vi "Slice Engine.vi"(8 "error in (no error)":errorcluster, 10 "Slice thickness  (mm)":dbl=150.0, 11 "System Parameters":T1={"Vibratome"={"Z Bottom [mm]"=0.0, "Pre Cut Dwell [s]"=1.0, "Blade Frequency [RPM]"=3000, "Slice Speed [mm/s]"=0.1, "Post Cut Dwell [s]"=4.0, "Ramp Time [s]"=0.5, "Start X [mm]"=80.5, "Start Y [mm]"=72.0, "Slice Length [mm]"=15.0, "Slice Axis"=enum."X Axis", "Controller VISA Ref"="COM3"}, "Table Stages"={"X Stage"={"Position"=0.0, "Is.Enabled?"=FALSE, "Is.Connected?"=FALSE, "Device SN"="45876060", "AccelerationMaximum"=50.0, "VelocityMaximum"=50.0, "Acceleration"=20.0, "Velocity"=20.0, "waitTimeout (ms)"=1000000, "Model"=enum."Thorlabs LTS", "Is.Homed?"=FALSE}, "Y Stage"={"Position"=0.0, "Is.Enabled?"=FALSE, "Is.Connected?"=FALSE, "Device SN"="45875512", "AccelerationMaximum"=50.0, "VelocityMaximum"=50.0, "Acceleration"=20.0, "Velocity"=20.0, "waitTimeout (ms)"=1000000, "Model"=enum."Thorlabs LTS", "Is.Homed?"=FALSE}, "Z Stage"={"Position"=0.0, "Is.Enabled?"=FALSE, "Is.Connected?"=FALSE, "Device SN"="49872414", "AccelerationMaximum"=50.0, "VelocityMaximum"=50.0, "Acceleration"=20.0, "Velocity"=20.0, "waitTimeout (ms)"=100000, "Model"=enum."Thorlabs MLJ", "Is.Homed?"=FALSE}}}) -> (0 "error out":errorcluster)   [LabVIEW 2017]
uses:
  Controls/System Parameters.ctl
  Hardware/Table Stage/Controls/Translation Stage Cluster.ctl
  Controls/Translation Stage Types.ctl
  Controls/Queue Manager Actions.ctl
  Controls/QueueNames.ctl
  Hardware/Table Stage/Controls/Motion Translation Module Control.ctl
  Controls/Set Get Controls.ctl
panel:
  in  "Last Slice?":bool
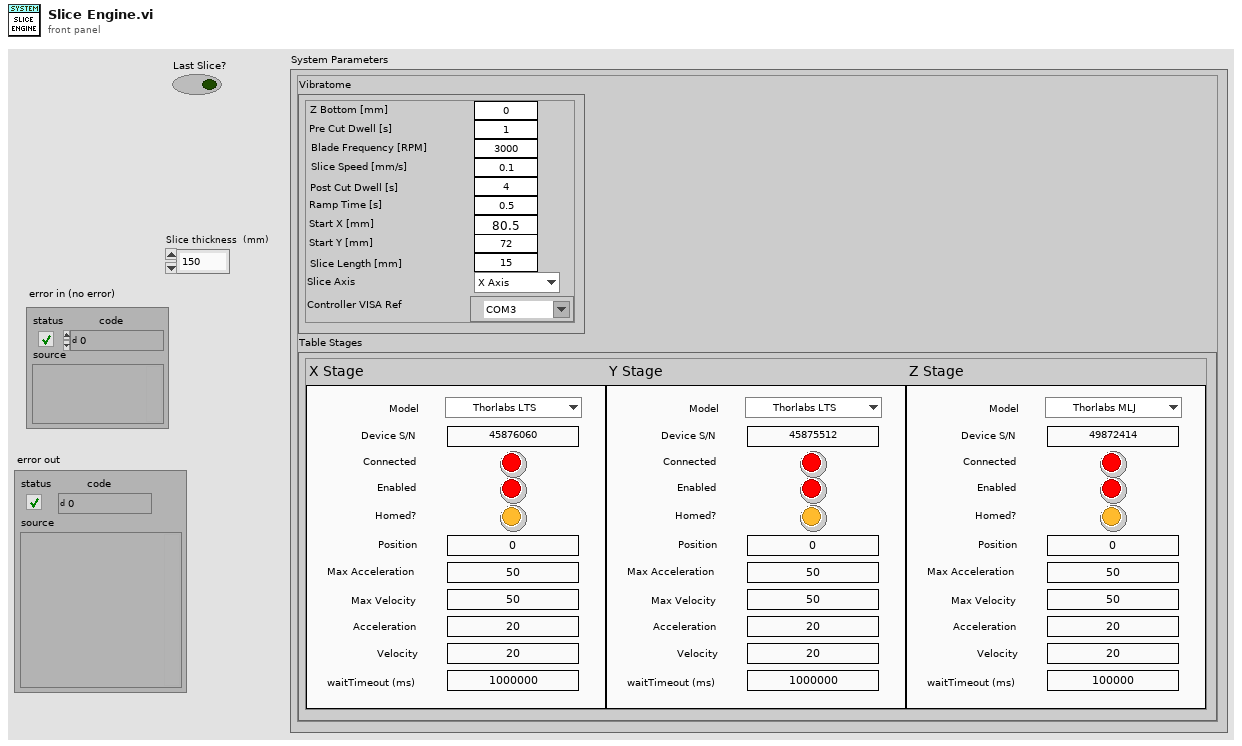
[diagram p1: front panel]
types:
  T1 = typedef "System Parameters.ctl" = cluster{"Vibratome":cluster{"Z Bottom [mm]":dbl, "Pre Cut Dwell [s]":dbl, "Blade Frequency [RPM]":u16, "Slice Speed [mm/s]":dbl, "Post Cut Dwell [s]":dbl, "Ramp Time [s]":dbl, "Start X [mm]":dbl, "Start Y [mm]":dbl, "Slice Length [mm]":dbl, "Slice Axis":enum16{"X Axis", "Y Axis", "Z Axis"}, "Controller VISA Ref":refnum<visa-resource-name>}, "Table Stages":cluster{"X Stage":T2, "Y Stage":T2, "Z Stage":T2}}
  T2 = typedef "Translation Stage Cluster.ctl" = cluster{"Position":dbl, "Is.Enabled?":bool, "Is.Connected?":bool, "Device SN":string, "AccelerationMaximum":dbl, "VelocityMaximum":dbl, "Acceleration":dbl, "Velocity":dbl, "waitTimeout (ms)":i32, "Model":T3, "Is.Homed?":bool}
  T3 = typedef "Translation Stage Types.ctl" = enum16{"None", "Thorlabs LTS", "Thorlabs MLJ"}
  T4 = typedef "QueueNames.ctl" = enum16{"Main GUI", "Main Scan Processor", "Main Display", "Main Table Stage GUI", "Main Table Stage Proc.", "Scan Engine", "Vibratome GUI", "Vibratome Processor", "Slice Engine"}
  T5 = typedef "Queue Manager Actions.ctl" = enum16{"Init", "Enqueue", "Enqueue All", "Preview Queue", "Dequeue", "Get Status", "Flush Queue", "Flush All Queues", "Release All Queues", "Release Queue", "Enqueue at Opposite End"}
  T6 = typedef "Set Get Controls.ctl" = enum16{"Set", "Get"}
  T7 = typedef "Motion Translation Module Control.ctl" = enum16{"Init", "Home", "Status", "Velocity/Accel", "Position", "Jog", "Stop", "Uninit", "Enable", "Disable"}
  T8 = enum16{"Set Configuration", "Get Configuration", "Enable Motor", "Disable Motor", "Get Status", "Open Session", "Close Session", "Set Limits", "Get Limits"}
  T9 = cluster{"Source for Velocity":enum16{"Interface", "Voltage (AI)", "PWM (AI)", "Current Target (AI)", "Current Target w/ Preset (AI)"}, "Mode":enum16{"Continuous", "Stepper Motor", "Analog Position Ctrl", "Encoder"}, "Target Velocity [RPM]":i16}
  T10 = typedef "MessagePacket.ctl" = cluster{"Message":string, "Parameter":variant}
  T11 = cluster{"X Stage":T2, "Y Stage":T2, "Z Stage":T2}
  T12 = enum16{"Left Button", "Center Button", "Right Button", "Window Close"}
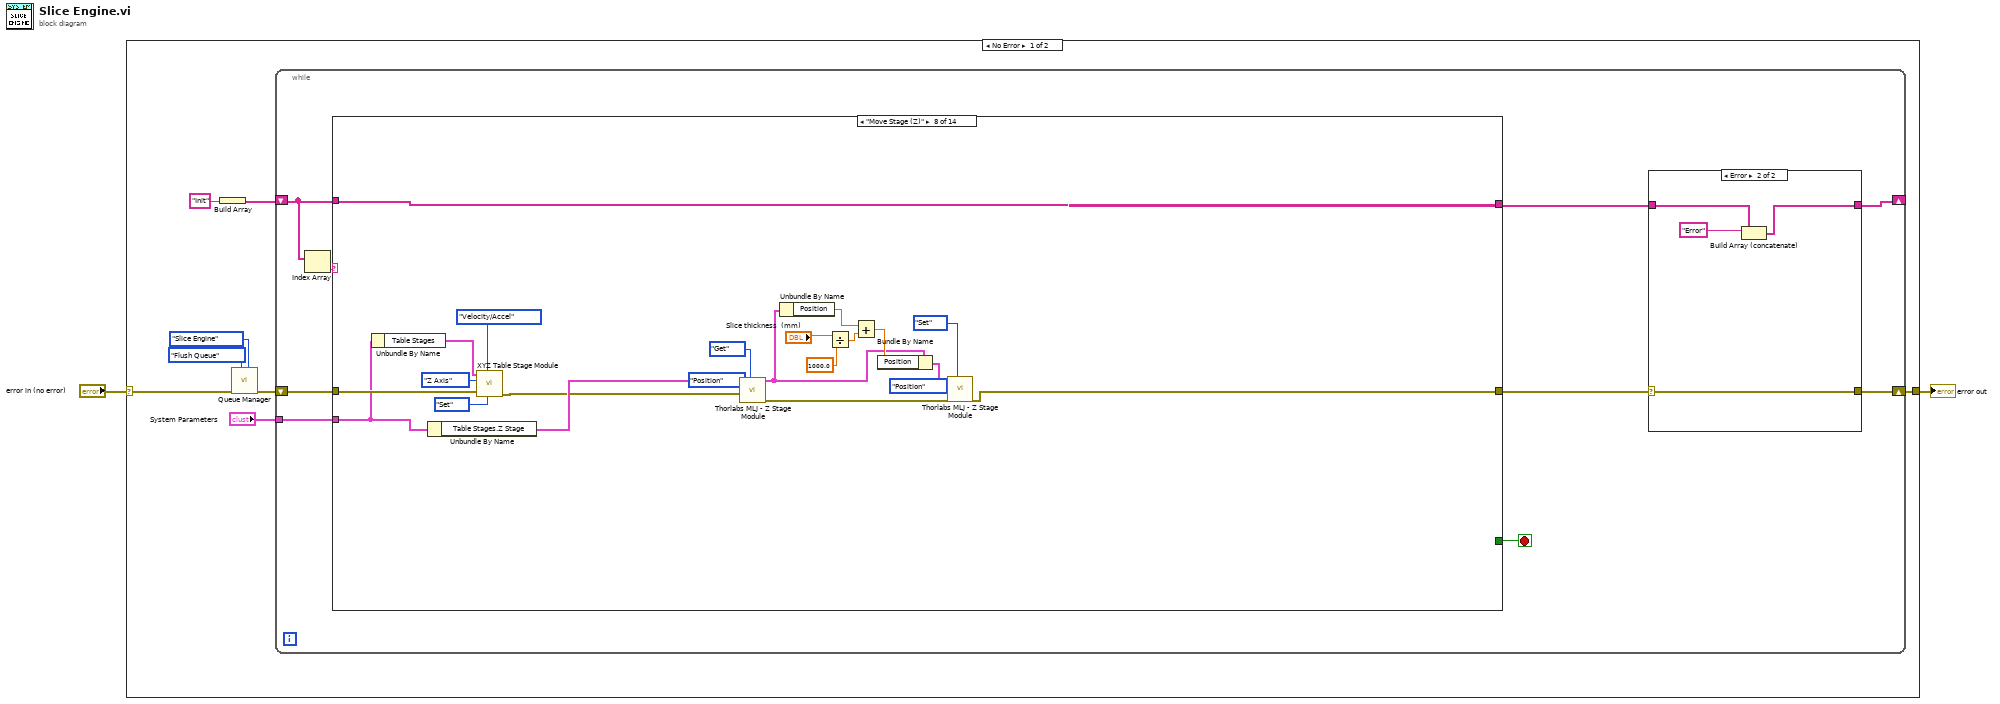
[diagram p0: block diagram]
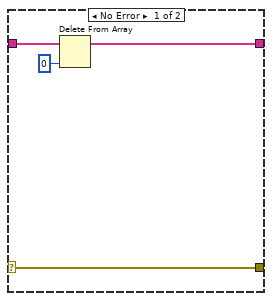
[diagram p2: hidden frame]
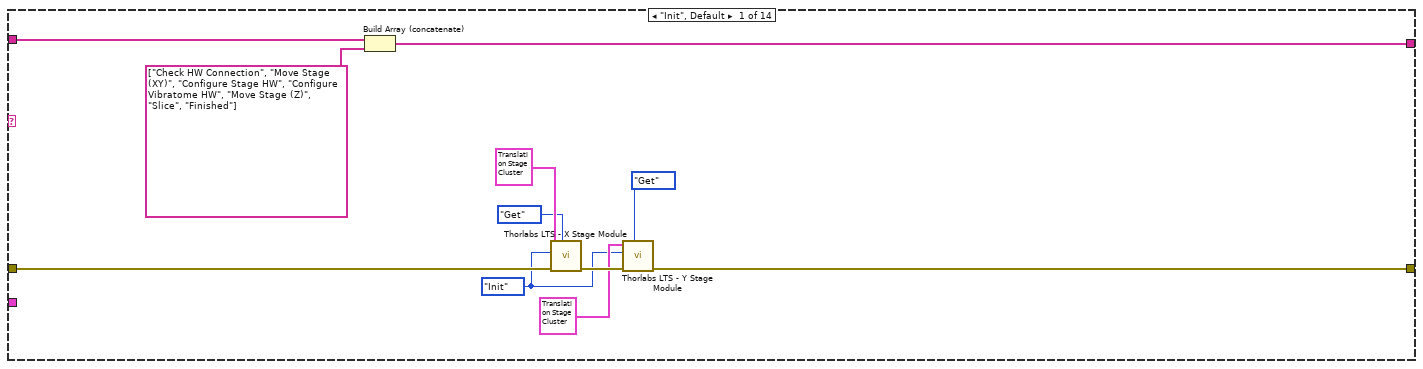
[diagram p3: hidden frame]
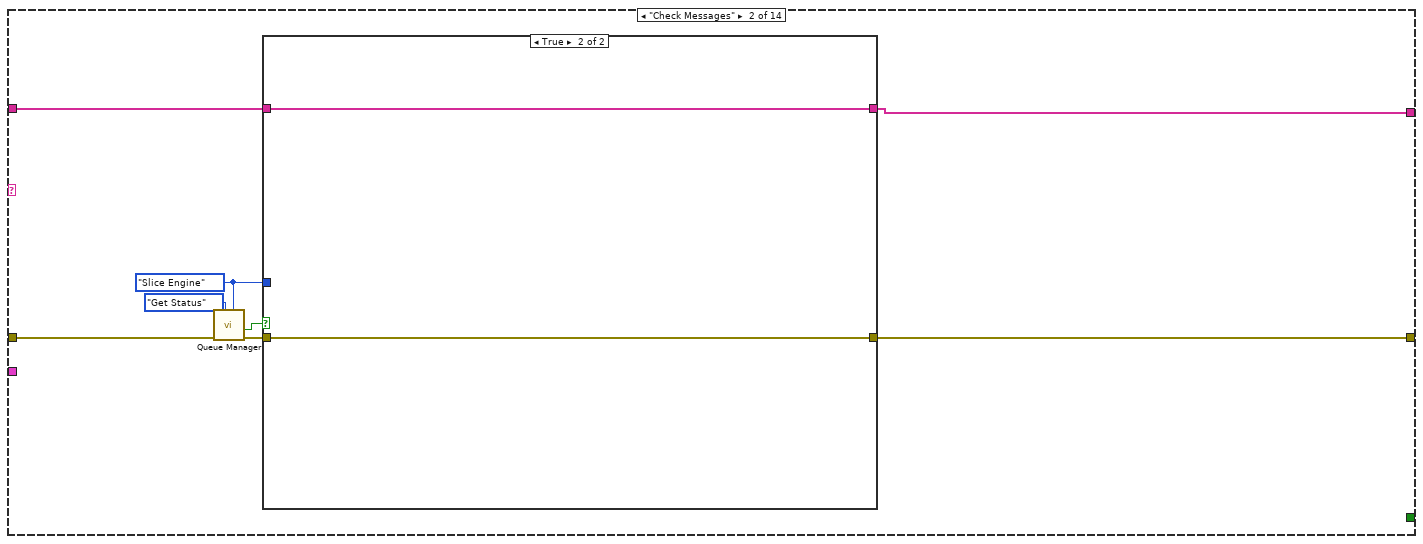
[diagram p4: hidden frame]
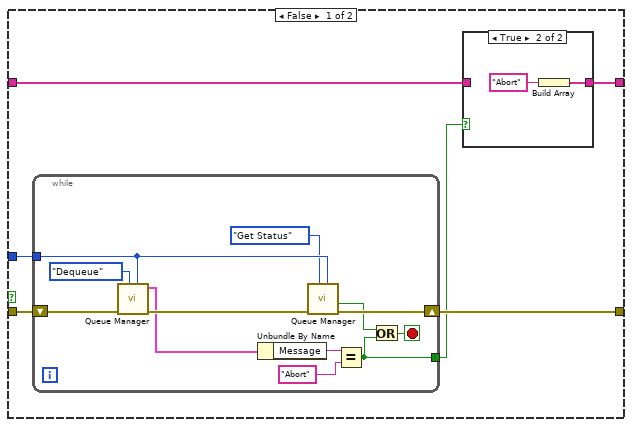
[diagram p5: hidden frame]
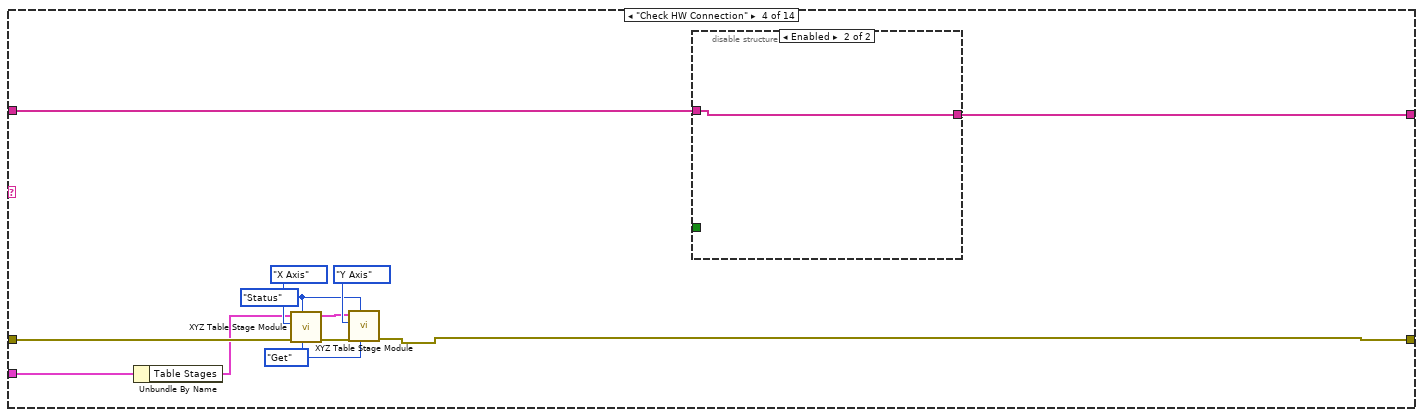
[diagram p8: hidden frame]
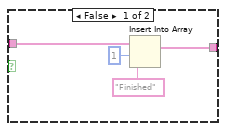
[diagram p10: hidden frame]
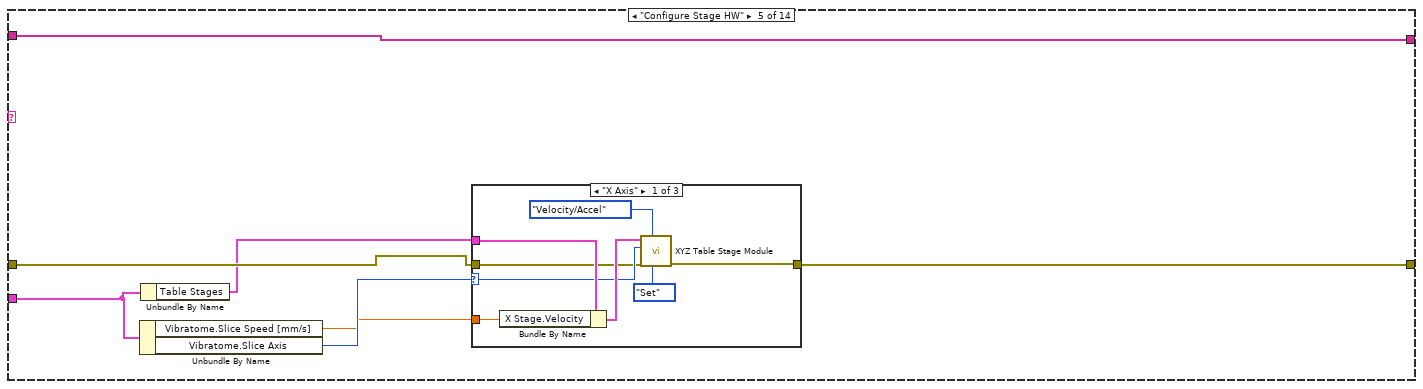
[diagram p11: hidden frame]
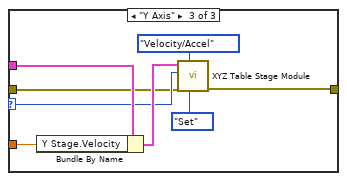
[diagram p13: hidden frame]
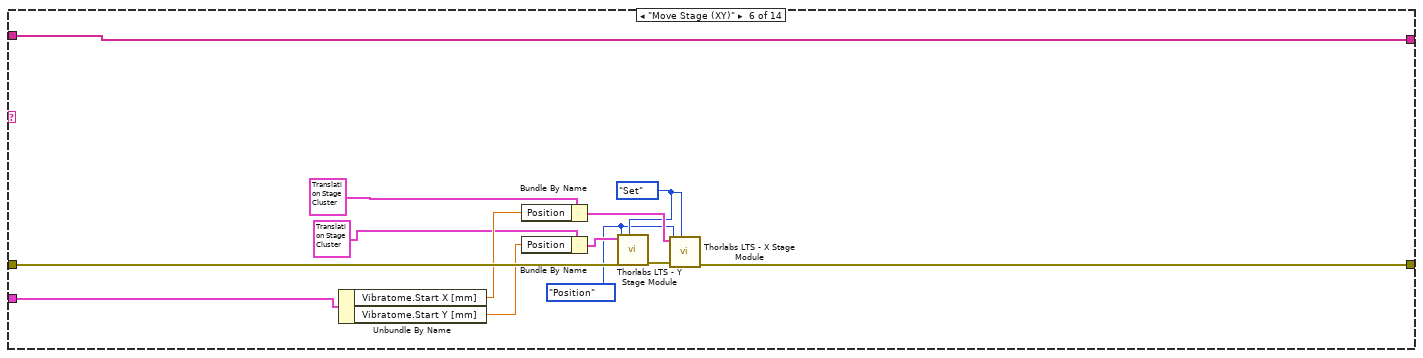
[diagram p14: hidden frame]
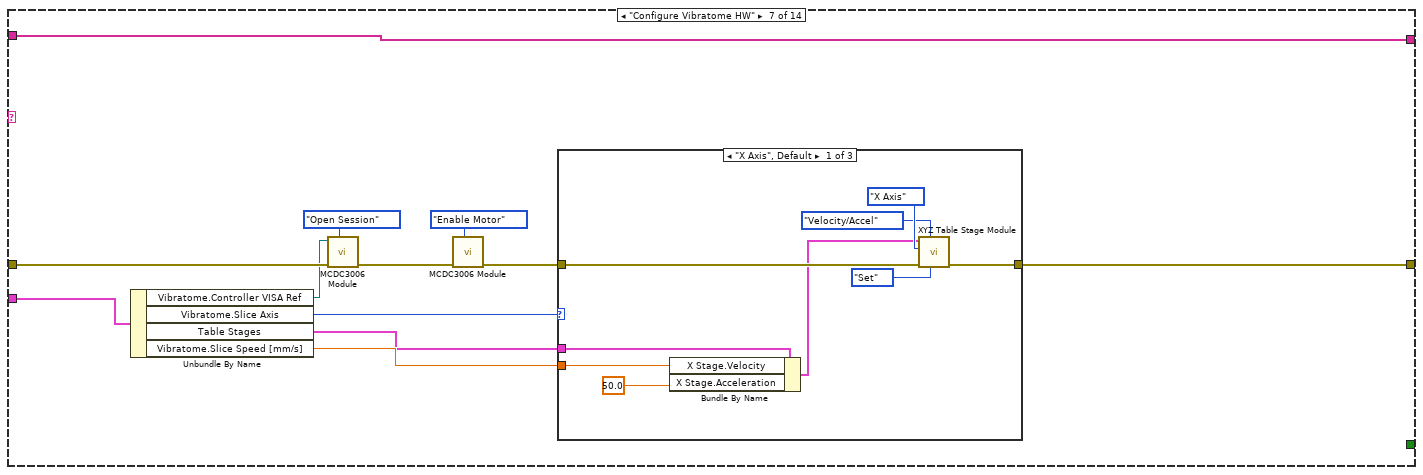
[diagram p15: hidden frame]
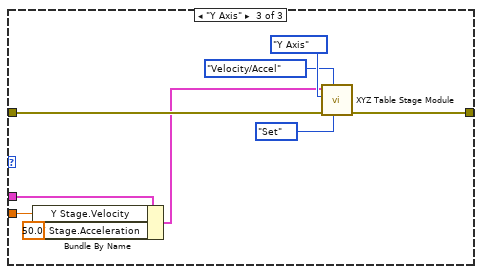
[diagram p17: hidden frame]
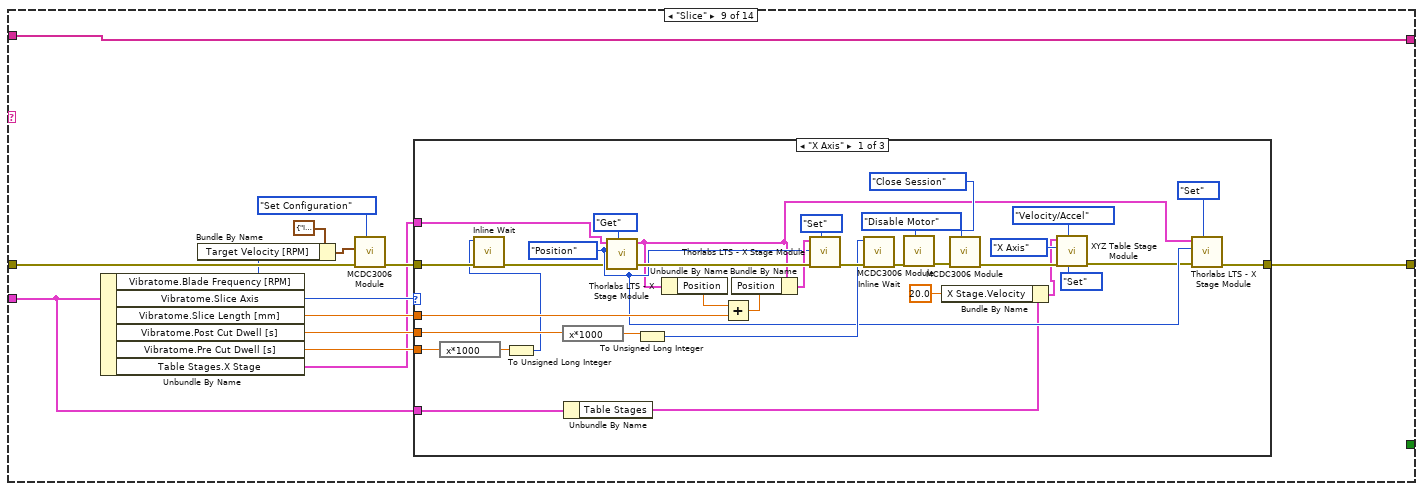
[diagram p18: hidden frame]
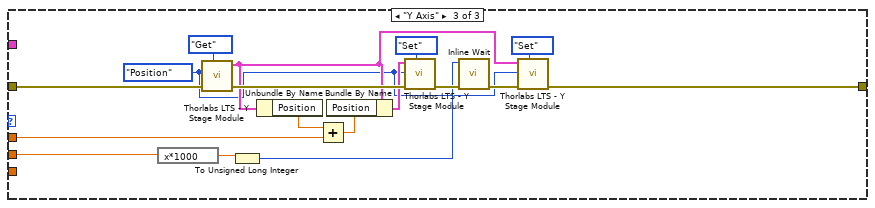
[diagram p20: hidden frame]
diagram:
  n1 = case shown="No Error" "error in (no error)" {
    selector: "error in (no error)" -> [w3 w392]
    tunnel: [w5 w392] -> w1
    frame No Error {
      n2 = Build Array("Init") -> (w6:string[])
      n3 = call "Queue Manager.vi"("Queue Name"=QueueNames."Slice Engine", "Action"=Queue_Manager_Actions."Flush Queue", "Error In"=w3) -> ("Error Out"=w9:errorcluster)  [unwired: 4 in, 4 out]
      n4 = while {
        shift-right: [w13] -> _
        shift-left: w6 -> [w12]
        shift-right: [w15] -> w5
        shift-left: w9 -> [w19]
        tunnel: "System Parameters" -> [w11]
        stop <- w17 stop-if-true
        n5 = Index Array(array=w12) -> (element=w18:string)  [unwired: 1 in]
        n6 = case shown="\"Move Stage (Z)\"" w18 {
          tunnel: w19 -> [w35 w46 w70 w83 w94 w129 w139 w167 w195 w249 w263 w267 w296 w365]
          tunnel: w12 -> [w38 w40 w71 w73 w99 w126 w141 w182 w194 w252 w260 w265 w297 w372]
          tunnel: [w37 w39 w71 w74 w99 w126 w141 w182 w194 w251 w261 w264 w297 w372] -> w14
          tunnel: [_ _ _ _ _ _ _ _ _ _ _ _ _ w371] -> w17
          tunnel: [w34 w41 w70 w72 w95 w128 w133 w176 w196 w249 w263 w268 w294 w363] -> w16
          tunnel: w11 -> [_ _ _ w82 w98 w127 w140 w163 w183 _ _ _ w295 w367]
          frame "Init", Default {
            w30 = Motion_Translation_Module_Control."Init" ("Action")
            n7 = Build Array (concatenate)(w38, string[] ["Check HW Connection", "Move Stage (XY)", "Configure Stage HW", "Configure Vibratome HW", "Move Stage (Z)", "Slice", "Finished"]) -> (w37:string[])
            n8 = call "Thorlabs LTS - X Stage Module.vi"("Set/Get"=Set_Get_Controls."Get", "Error In"=w35, "Action"=w30, "Cluster In"=T2 {"Position"=0.0, "Is.Enabled?"=TRUE, "Is.Connected?"=FALSE, "Device SN"="45876060", "AccelerationMaximum"=0.0, "VelocityMaximum"=0.0, "Acceleration"=0.0, "Velocity"=0.0, "waitTimeout (ms)"=10000, "Model"=enum."None", "Is.Homed?"=FALSE}) -> ("Error Out"=w33:errorcluster)  [unwired: 6 in, 1 out]
            n9 = call "Thorlabs LTS - Y Stage Module.vi"("Set/Get"=Set_Get_Controls."Get", "Error In"=w33, "Action"=w30, "Cluster In"=T2 {"Position"=0.0, "Is.Enabled?"=TRUE, "Is.Connected?"=FALSE, "Device SN"="45875512", "AccelerationMaximum"=0.0, "VelocityMaximum"=0.0, "Acceleration"=0.0, "Velocity"=0.0, "waitTimeout (ms)"=10000, "Model"=enum."None", "Is.Homed?"=FALSE}) -> ("Error Out"=w34:errorcluster)  [unwired: 6 in, 1 out]
          }
          frame "Check Messages" {
            w42 = QueueNames."Slice Engine" ("Queue Name")
            n10 = call "Queue Manager.vi"("Queue Name"=w42, "Action"=Queue_Manager_Actions."Get Status", "Error In"=w46) -> ("Error Out"=w43:errorcluster, "Empty?"=w44:bool)  [unwired: 4 in, 3 out]
            n11 = case shown="True" w44 {
              tunnel: w43 -> [w52 w68]
              tunnel: w42 -> [w51 _]
              tunnel: [w50 w68] -> w41
              tunnel: w40 -> [w48 w69]
              tunnel: [w47 w69] -> w39
              frame False {
                n12 = while {
                  tunnel: w51 -> [w63]
                  shift-right: [w64] -> w50
                  shift-left: w52 -> [w67]
                  tunnel: [w56] -> w49
                  stop <- w57 stop-if-true
                  n13 = call "Queue Manager.vi"("Queue Name"=w63, "Action"=Queue_Manager_Actions."Dequeue", "Error In"=w67) -> ("Error Out"=w65:errorcluster, "Message Packet [Out]"=w61:T10)  [unwired: 4 in, 3 out]
                  n14 = Unbundle By Name(w61) -> ("Message"=w60:string)
                  n15 = call "Queue Manager.vi"("Queue Name"=w63, "Action"=Queue_Manager_Actions."Get Status", "Error In"=w65) -> ("Error Out"=w64:errorcluster, "Empty?"=w58:bool)  [unwired: 4 in, 3 out]
                  n16 = Equal?(x=w60, y="Abort") -> (x = y?=w56:bool)
                  n17 = Or(x=w58, y=w56) -> (x .or. y?=w57:bool)
                }
                n18 = case shown="True" w49 {
                  tunnel: w48 -> [w53 _]
                  tunnel: [w53 w54] -> w47
                  frame False {
                  }
                  frame True {
                    n19 = Build Array("Abort") -> (w54:string[])
                  }
                }
              }
              frame True {
              }
            }
          }
          frame "Load Parameters" {
          }
          frame "Check HW Connection" {
            w77 = Set_Get_Controls."Get" ("Set/Get")
            w78 = Motion_Translation_Module_Control."Status" ("Action")
            n20 = Unbundle By Name(w82) -> ("Table Stages"=w76:T11)
            n21 = call "XYZ Table Stage Module.vi"("Set/Get"=w77, "Action"=w78, "Error In"=w83, "Axis"=enum16{"X Axis", "Y Axis", "Z Axis"}."X Axis", "Table Stages"=w76) -> ("Error Out"=w81:errorcluster, "Table Stages Out"=w75:T11)  [unwired: 5 in]
            n22 = call "XYZ Table Stage Module.vi"("Set/Get"=w77, "Action"=w78, "Error In"=w81, "Axis"=enum16{"X Axis", "Y Axis", "Z Axis"}."Y Axis", "Table Stages"=w75) -> ("Error Out"=w72:errorcluster)  [unwired: 5 in, 1 out]
            n23 = disable-structure shown="Enabled" {
              disable-tunnel: [w86 w92] -> w74
              disable-tunnel: w73 -> [w85 w92]
              disable-tunnel: _ -> [w84 _]
              frame Disabled {
                n24 = case "Checks Stage Status OK" shown="True" w84 {
                  tunnel: [w90 w91] -> w86
                  tunnel: w85 -> [w89 w91]
                  frame False {
                    n25 = Insert Into Array(array=w89, index=1, new element="Finished" ("new element/subarray")) -> (w90:string[])
                  }
                  frame True {
                  }
                }
              }
              frame Enabled {
              }
            }
          }
          frame "Configure Stage HW" {
            n26 = Unbundle By Name(w98) -> ("Vibratome.Slice Speed [mm/s]"=w96:dbl, "Vibratome.Slice Axis"=w97:enum16{"X Axis", "Y Axis", "Z Axis"})
            n27 = Unbundle By Name(w98) -> ("Table Stages"=w93:T11)
            n28 = case shown="\"X Axis\"" w97 {
              selector: w97 -> [w104 _ w113]
              tunnel: w96 -> [w107 _ w116]
              tunnel: w93 -> [w106 _ w115]
              tunnel: w94 -> [w103 w108 w112]
              tunnel: [w102 w108 w111] -> w95
              frame "X Axis" {
                n29 = Bundle By Name(cluster=w106, "X Stage.Velocity"=w107) -> (w105:T11)
                n30 = call "XYZ Table Stage Module.vi"("Set/Get"=Set_Get_Controls."Set", "Action"=Motion_Translation_Module_Control."Velocity/Accel", "Error In"=w103, "Axis"=w104, "Table Stages"=w105) -> ("Error Out"=w102:errorcluster)  [unwired: 5 in, 1 out]
              }
              frame "Z Axis" {
              }
              frame "Y Axis" {
                n31 = Bundle By Name(cluster=w115, "Y Stage.Velocity"=w116) -> (w114:T11)
                n32 = call "XYZ Table Stage Module.vi"("Set/Get"=Set_Get_Controls."Set", "Action"=Motion_Translation_Module_Control."Velocity/Accel", "Error In"=w112, "Axis"=w113, "Table Stages"=w114) -> ("Error Out"=w111:errorcluster)  [unwired: 5 in, 1 out]
              }
            }
          }
          frame "Move Stage (XY)" {
            w119 = Motion_Translation_Module_Control."Position" ("Action")
            w120 = Set_Get_Controls."Set" ("Set/Get")
            n33 = Unbundle By Name(w127) -> ("Vibratome.Start X [mm]"=w122:dbl, "Vibratome.Start Y [mm]"=w121:dbl)
            n34 = Bundle By Name(cluster=T2 {"Position"=0.0, "Is.Enabled?"=TRUE, "Is.Connected?"=FALSE, "Device SN"="45876060", "AccelerationMaximum"=50.0, "VelocityMaximum"=50.0, "Acceleration"=50.0, "Velocity"=50.0, "waitTimeout (ms)"=10000000, "Model"=enum."Thorlabs LTS", "Is.Homed?"=FALSE} ("Cluster In"), "Position"=w122) -> (w125:T2)
            n35 = Bundle By Name(cluster=T2 {"Position"=0.0, "Is.Enabled?"=TRUE, "Is.Connected?"=FALSE, "Device SN"="45875512", "AccelerationMaximum"=50.0, "VelocityMaximum"=50.0, "Acceleration"=50.0, "Velocity"=50.0, "waitTimeout (ms)"=10000000, "Model"=enum."Thorlabs LTS", "Is.Homed?"=FALSE} ("Cluster In"), "Position"=w121) -> (w123:T2)
            n36 = call "Thorlabs LTS - Y Stage Module.vi"("Set/Get"=w120, "Error In"=w129, "Action"=w119, "Cluster In"=w123) -> ("Error Out"=w117:errorcluster)  [unwired: 6 in, 1 out]
            n37 = call "Thorlabs LTS - X Stage Module.vi"("Set/Get"=w120, "Error In"=w117, "Action"=w119, "Cluster In"=w125) -> ("Error Out"=w128:errorcluster)  [unwired: 6 in, 1 out]
          }
          frame "Configure Vibratome HW" {
            n38 = Unbundle By Name(w140) -> ("Vibratome.Controller VISA Ref"=w137:refnum<visa-resource-name>, "Vibratome.Slice Axis"=w132:enum16{"X Axis", "Y Axis", "Z Axis"}, "Table Stages"=w130:T11, "Vibratome.Slice Speed [mm/s]"=w131:dbl)
            n39 = call "MCDC3006 Module.vi"("Actions"=T8."Open Session", "Error In"=w139, "VISA resource name"=w137) -> ("Error Out"=w135:errorcluster)  [unwired: 4 in, 4 out]
            n40 = call "MCDC3006 Module.vi"("Actions"=T8."Enable Motor", "Error In"=w135) -> ("Error Out"=w134:errorcluster)  [unwired: 5 in, 4 out]
            n41 = case shown="\"X Axis\", Default" w132 {
              tunnel: [w150 w151 w160] -> w133
              tunnel: w134 -> [w145 w151 w156]
              tunnel: w131 -> [w146 _ w155]
              tunnel: w130 -> [w143 _ w154]
              frame "X Axis", Default {
                n42 = Bundle By Name(cluster=w143, "X Stage.Velocity"=w146, "X Stage.Acceleration"=50.0 ("Acceleration")) -> (w142:T11)
                n43 = call "XYZ Table Stage Module.vi"("Set/Get"=Set_Get_Controls."Set", "Action"=Motion_Translation_Module_Control."Velocity/Accel", "Error In"=w145, "Axis"=enum16{"X Axis", "Y Axis", "Z Axis"}."X Axis", "Table Stages"=w142) -> ("Error Out"=w150:errorcluster)  [unwired: 5 in, 1 out]
              }
              frame "Z Axis" {
              }
              frame "Y Axis" {
                n44 = Bundle By Name(cluster=w154, "Y Stage.Velocity"=w155, "Y Stage.Acceleration"=50.0 ("Acceleration")) -> (w152:T11)
                n45 = call "XYZ Table Stage Module.vi"("Set/Get"=Set_Get_Controls."Set", "Action"=Motion_Translation_Module_Control."Velocity/Accel", "Error In"=w156, "Axis"=enum16{"X Axis", "Y Axis", "Z Axis"}."Y Axis", "Table Stages"=w152) -> ("Error Out"=w160:errorcluster)  [unwired: 5 in, 1 out]
              }
            }
          }
          frame "Move Stage (Z)" {
            n46 = Unbundle By Name(w163) -> ("Table Stages"=w162:T11)
            n47 = Unbundle By Name(w163) -> ("Table Stages.Z Stage"=w172:T2)
            n48 = call "XYZ Table Stage Module.vi"("Set/Get"=Set_Get_Controls."Set", "Action"=Motion_Translation_Module_Control."Velocity/Accel", "Error In"=w167, "Axis"=enum16{"X Axis", "Y Axis", "Z Axis"}."Z Axis", "Table Stages"=w162) -> ("Error Out"=w166:errorcluster)  [unwired: 5 in, 1 out]
            n49 = call "Thorlabs MLJ - Z Stage Module.vi"("Set/Get"=Set_Get_Controls."Get", "Error In"=w166, "Action"=Motion_Translation_Module_Control."Position", "Cluster In"=w172) -> ("Error Out"=w178:errorcluster, "Cluster Out"=w174:T2)  [unwired: 6 in]
            n50 = Unbundle By Name(w174) -> ("Position"=w171:dbl)
            n51 = Divide(x="Slice thickness  (mm)", y=1000.0) -> (x/y=w170:dbl)
            n52 = Add(x=w171, y=w170) -> (x+y=w175:dbl)
            n53 = Bundle By Name(cluster=w174, "Position"=w175) -> (w173:T2)
            n54 = call "Thorlabs MLJ - Z Stage Module.vi"("Set/Get"=Set_Get_Controls."Set", "Error In"=w178, "Action"=Motion_Translation_Module_Control."Position", "Cluster In"=w173) -> ("Error Out"=w176:errorcluster)  [unwired: 6 in, 1 out]
          }
          frame "Slice" {
            n55 = Unbundle By Name(w183) -> ("Vibratome.Blade Frequency [RPM]"=w188:u16, "Vibratome.Slice Axis"=w193:enum16{"X Axis", "Y Axis", "Z Axis"}, "Vibratome.Slice Length [mm]"=w192:dbl, "Vibratome.Post Cut Dwell [s]"=w186:dbl, "Vibratome.Pre Cut Dwell [s]"=w185:dbl, "Table Stages.X Stage"=w184:T2)
            n56 = Bundle By Name(cluster=T9 {"Source for Velocity"=enum."Interface", "Mode"=enum."Continuous", "Target Velocity [RPM]"=0} ("Configuration [In]"), "Target Velocity [RPM]"=w188) -> (w187:T9)
            n57 = call "MCDC3006 Module.vi"("Actions"=T8."Set Configuration", "Error In"=w195, "Configuration [In]"=w187) -> ("Error Out"=w191:errorcluster)  [unwired: 4 in, 4 out]
            n58 = case shown="\"X Axis\"" w193 {
              tunnel: w191 -> [w230 w231 w248]
              tunnel: [w218 w231 w235] -> w196
              tunnel: w192 -> [w224 _ w242]
              tunnel: w186 -> [w221 _ w238]
              tunnel: w185 -> [w214 _ _]
              tunnel: w184 -> [w209 _ _]
              tunnel: w183 -> [w199 _ _]
              frame "X Axis" {
                w216 = Motion_Translation_Module_Control."Position" ("Action")
                n59 = expression code="x*1000"(w214) -> (w213:dbl)
                n60 = To Unsigned Long Integer(number=w213) -> (unsigned 32bit integer=w212:u32)
                n61 = call "Inline Wait.vi"("Error In"=w230, "milliseconds to wait"=w212) -> ("Error Out"=w215:errorcluster)  [unwired: 9 in]
                n62 = expression code="x*1000"(w221) -> (w220:dbl)
                n63 = Unbundle By Name(w199) -> ("Table Stages"=w198:T11)
                n64 = call "Thorlabs LTS - X Stage Module.vi"("Set/Get"=Set_Get_Controls."Get", "Error In"=w215, "Action"=w216, "Cluster In"=w209) -> ("Error Out"=w229:errorcluster, "Cluster Out"=w205:T2)  [unwired: 6 in]
                n65 = To Unsigned Long Integer(number=w220) -> (unsigned 32bit integer=w219:u32)
                n66 = Unbundle By Name(w205) -> ("Position"=w225:dbl)
                n67 = Add(x=w225, y=w224) -> (x+y=w223:dbl)
                n68 = Bundle By Name(cluster=w205, "Position"=w223) -> (w222:T2)
                n69 = call "Thorlabs LTS - X Stage Module.vi"("Set/Get"=Set_Get_Controls."Set", "Error In"=w229, "Action"=w216, "Cluster In"=w222) -> ("Error Out"=w227:errorcluster)  [unwired: 6 in, 1 out]
                n70 = call "Inline Wait.vi"("Error In"=w227, "milliseconds to wait"=w219) -> ("Error Out"=w211:errorcluster)  [unwired: 9 in]
                n71 = call "MCDC3006 Module.vi"("Actions"=T8."Disable Motor", "Error In"=w211) -> ("Error Out"=w207:errorcluster)  [unwired: 5 in, 4 out]
                n72 = Bundle By Name(cluster=w198, "X Stage.Velocity"=20.0 ("Velocity")) -> (w197:T11)
                n73 = call "MCDC3006 Module.vi"("Actions"=T8."Close Session", "Error In"=w207) -> ("Error Out"=w204:errorcluster)  [unwired: 5 in, 4 out]
                n74 = call "XYZ Table Stage Module.vi"("Set/Get"=Set_Get_Controls."Set", "Action"=Motion_Translation_Module_Control."Velocity/Accel", "Error In"=w204, "Axis"=enum16{"X Axis", "Y Axis", "Z Axis"}."X Axis", "Table Stages"=w197) -> ("Error Out"=w203:errorcluster)  [unwired: 5 in, 1 out]
                n75 = call "Thorlabs LTS - X Stage Module.vi"("Set/Get"=Set_Get_Controls."Set", "Error In"=w203, "Action"=w216, "Cluster In"=w205) -> ("Error Out"=w218:errorcluster)  [unwired: 6 in, 1 out]
              }
              frame "Z Axis" {
              }
              frame "Y Axis" {
                w232 = Motion_Translation_Module_Control."Position" ("Action")
                n76 = expression code="x*1000"(w238) -> (w237:dbl)
                n77 = call "Thorlabs LTS - Y Stage Module.vi"("Set/Get"=Set_Get_Controls."Get", "Error In"=w248, "Action"=w232) -> ("Error Out"=w247:errorcluster, "Cluster Out"=w233:T2)  [unwired: 7 in]
                n78 = To Unsigned Long Integer(number=w237) -> (unsigned 32bit integer=w236:u32)
                n79 = Unbundle By Name(w233) -> ("Position"=w243:dbl)
                n80 = Add(x=w243, y=w242) -> (x+y=w241:dbl)
                n81 = Bundle By Name(cluster=w233, "Position"=w241) -> (w240:T2)
                n82 = call "Thorlabs LTS - Y Stage Module.vi"("Set/Get"=Set_Get_Controls."Set", "Error In"=w247, "Action"=w232, "Cluster In"=w240) -> ("Error Out"=w245:errorcluster)  [unwired: 6 in, 1 out]
                n83 = call "Inline Wait.vi"("Error In"=w245, "milliseconds to wait"=w236) -> ("Error Out"=w239:errorcluster)  [unwired: 9 in]
                n84 = call "Thorlabs LTS - Y Stage Module.vi"("Set/Get"=Set_Get_Controls."Set", "Error In"=w239, "Action"=w232, "Cluster In"=w233) -> ("Error Out"=w235:errorcluster)  [unwired: 6 in, 1 out]
              }
            }
          }
          frame "Next Slice" {
            n85 = case shown="False" "Last Slice?" {
              tunnel: w252 -> [w256 w257]
              tunnel: [w255 w257] -> w251
              frame False {
                n86 = Insert Into Array(array=w256, index=1, new element=string[] ["Move Stage (Z)", "Slice", "Next Slice"]) -> (w255:string[])
              }
              frame True {
              }
            }
          }
          frame "Abort" {
            n87 = Insert Into Array(array=w260, index=1, new element #1="Uninit", new element #2="Finished") -> (w261:string[])
          }
          frame "Error" {
            n88 = control-ref of="This VI"() -> (w278:refnum<vi>)
            n89 = property class="VI"(reference=w278) -> ("Name"=w281:string, "Callers"=w283:string[])  [unwired: 1 in, 2 out]
            n90 = Unbundle(w267) -> ("code"=w277:i32, "source"=w276:string)  [unwired: 1 out]
            n91 = Array To Spreadsheet String(delimiter (Tab)=">", array=w283, 3:"%s" ("format string")) -> (spreadsheet string=w282:string)
            n92 = Format Into String(format string="VI Name: %s\nCallers: %s\nError Code: %d\nError Message: %s", initial string="The following error occurred:\n" ("message"), w281, w282, w277, w276) -> (resulting string=w275:string, error out=w269:errorcluster)  [unwired: 1 in]
            n93 = call <vilib>:"Clear Errors.vi"("error in (no error)"=w269) -> ()  [unwired: 5 in, 2 out]
            n94 = call <vilib>:"Three Button Dialog.vi"("Allow user to close window? (TRUE)"=FALSE, "Window Title (\"\")"="Error" ("Window Title (\"\")"), "Right Button Text (\"Cancel\")"="Abort" ("Right Button Text (\"Cancel\")"), "Center Button Text (\"No\")"="Retry" ("Center Button Text (\"No\")"), "Left Button Text (\"Yes\")"="Continue" ("Left Button Text (\"Yes\")"), "message"=w275) -> ("Which Button?"=w266:T12)  [unwired: 5 in]
            n95 = case shown="\"Right Button\"" w266 {
              tunnel: w265 -> [w288 w292 w293]
              tunnel: [w287 w291 w293] -> w264
              frame "Left Button", Default {
                # "Continue"
                n96 = Delete From Array(array=w288, index=0) -> (array with subset deleted=w287:string[])  [unwired: 1 in, 1 out]
              }
              frame "Right Button" {
                # "Abort"
                n97 = Insert Into Array(array=w292, index=1, new element="Abort") -> (w291:string[])
              }
              frame "Center Button" {
                # "Retry"
              }
            }
            n98 = call <vilib>:"Clear Errors.vi"("error in (no error)"=w267) -> ("error out"=w268:errorcluster)  [unwired: 5 in, 1 out]
          }
          frame "Uninit" {
            n99 = disable-structure shown="Enabled" {
              disable-tunnel: w296 -> [w301 w362]
              disable-tunnel: w295 -> [w300 _]
              disable-tunnel: [w299 w355] -> w294
              frame Enabled {
                n100 = for {
                  N: 4 -> [_]
                  tunnel: [w307] -> w302 mode=indexing
                  tunnel: Motion_Translation_Module_Control."Uninit" ("Action") -> [w306]
                  tunnel: w301 -> [w305]
                  tunnel: w300 -> [w304]
                  i -> [w308]
                  n101 = case shown="3" w308 {
                    tunnel: [w314 w326 w340 w349] -> w307
                    tunnel: w305 -> [w313 w325 w339 w349]
                    tunnel: w306 -> [w312 w324 w338 _]
                    tunnel: w304 -> [w311 w323 w337 _]
                    frame 0, Default {
                      # "X Stage"
                      n102 = Unbundle By Name(w311) -> ("Table Stages.X Stage.Model"=w310:T3, "Table Stages.X Stage"=w309:T2)
                      n103 = case shown="\"Thorlabs LTS\"" w310 {
                        tunnel: [w315 w320] -> w314
                        tunnel: w313 -> [w315 w319]
                        tunnel: w312 -> [_ w318]
                        tunnel: w309 -> [_ w316]
                        frame "None", Default {
                        }
                        frame "Thorlabs LTS" {
                          n104 = call "Thorlabs LTS - X Stage Module.vi"("Set/Get"=Set_Get_Controls."Set", "Error In"=w319, "Action"=w318, "Cluster In"=w316) -> ("Error Out"=w320:errorcluster)  [unwired: 6 in, 1 out]
                        }
                      }
                    }
                    frame 1 {
                      # "Y Stage"
                      n105 = Unbundle By Name(w323) -> ("Table Stages.Y Stage.Model"=w322:T3, "Table Stages.Y Stage.Device SN"=w321:string)
                      n106 = case shown="\"Thorlabs LTS\"" w322 {
                        tunnel: [w327 w334] -> w326
                        tunnel: w325 -> [w327 w333]
                        tunnel: w324 -> [_ w332]
                        tunnel: w321 -> [_ w330]
                        frame "None", Default {
                        }
                        frame "Thorlabs LTS" {
                          n107 = Bundle By Name(cluster=T2 {"Position"=0.0, "Is.Enabled?"=TRUE, "Is.Connected?"=FALSE, "Device SN"="45876539", "AccelerationMaximum"=0.0, "VelocityMaximum"=0.0, "Acceleration"=0.0, "Velocity"=0.0, "waitTimeout (ms)"=0, "Model"=enum."Thorlabs LTS", "Is.Homed?"=FALSE} ("Cluster In"), "Device SN"=w330) -> (w329:T2)
                          n108 = call "Thorlabs LTS - Y Stage Module.vi"("Set/Get"=Set_Get_Controls."Set", "Error In"=w333, "Action"=w332, "Cluster In"=w329) -> ("Error Out"=w334:errorcluster)  [unwired: 6 in, 1 out]
                        }
                      }
                    }
                    frame 2 {
                      # "Z Stage"
                      n109 = Unbundle By Name(w337) -> ("Table Stages.Z Stage.Model"=w336:T3, "Table Stages.Z Stage.Device SN"=w335:string)
                      n110 = case shown="\"Thorlabs MLJ\"" w336 {
                        tunnel: [w341 w348] -> w340
                        tunnel: w339 -> [w341 w347]
                        tunnel: w338 -> [_ w346]
                        tunnel: w335 -> [_ w344]
                        frame "None", Default {
                        }
                        frame "Thorlabs MLJ" {
                          n111 = Bundle By Name(cluster=T2 {"Position"=0.0, "Is.Enabled?"=TRUE, "Is.Connected?"=FALSE, "Device SN"="45876539", "AccelerationMaximum"=0.0, "VelocityMaximum"=0.0, "Acceleration"=0.0, "Velocity"=0.0, "waitTimeout (ms)"=0, "Model"=enum."Thorlabs MLJ", "Is.Homed?"=FALSE} ("Cluster In"), "Device SN"=w344) -> (w343:T2)
                          n112 = call "Thorlabs MLJ - Z Stage Module.vi"("Set/Get"=Set_Get_Controls."Set", "Error In"=w347, "Action"=w346, "Cluster In"=w343) -> ("Error Out"=w348:errorcluster)  [unwired: 6 in, 1 out]
                        }
                      }
                    }
                    frame 3 {
                      # "Vibratome Motor"
                    }
                  }
                }
                n113 = Merge Errors(w302) -> (w299:errorcluster)
              }
              frame Disabled {
                w350 = Set_Get_Controls."Set" ("Set/Get")
                w354 = Motion_Translation_Module_Control."Uninit" ("Action")
                n114 = call "XYZ Table Stage Module.vi"("Set/Get"=w350, "Action"=w354, "Error In"=w362, "Axis"=enum16{"X Axis", "Y Axis", "Z Axis"}."X Axis") -> ("Error Out"=w361:errorcluster)  [unwired: 6 in, 1 out]
                n115 = call "XYZ Table Stage Module.vi"("Set/Get"=w350, "Action"=w354, "Error In"=w361, "Axis"=enum16{"X Axis", "Y Axis", "Z Axis"}."Y Axis") -> ("Error Out"=w360:errorcluster)  [unwired: 6 in, 1 out]
                n116 = call "XYZ Table Stage Module.vi"("Set/Get"=w350, "Action"=w354, "Error In"=w360, "Axis"=enum16{"X Axis", "Y Axis", "Z Axis"}."Z Axis") -> ("Error Out"=w357:errorcluster)  [unwired: 6 in, 1 out]
                n117 = call "MCDC3006 Module.vi"("Actions"=T8."Disable Motor", "Error In"=w357) -> ("Error Out"=w356:errorcluster)  [unwired: 5 in, 4 out]
                n118 = call "MCDC3006 Module.vi"("Actions"=T8."Close Session", "Error In"=w356) -> ("Error Out"=w355:errorcluster)  [unwired: 5 in, 4 out]
              }
            }
          }
          frame "Finished" {
            n119 = Unbundle By Name(w367) -> ("Table Stages"=w368:T11)
            n120 = Unbundle By Name(w367) -> ("Table Stages.X Stage.Velocity"=w369:dbl, "Vibratome.Slice Axis"=w366:enum16{"X Axis", "Y Axis", "Z Axis"})
            n121 = case shown="\"Y Axis\"" w366 {
              selector: w366 -> [w381 _ w390]
              tunnel: w369 -> [w382 _ w391]
              tunnel: w368 -> [w376 _ w385]
              tunnel: [w380 w383 w389] -> w364
              tunnel: w365 -> [w377 w383 w386]
              frame "X Axis" {
                n122 = Bundle By Name(cluster=w376, "X Stage.Velocity"=w382) -> (w375:T11)
                n123 = call "XYZ Table Stage Module.vi"("Set/Get"=Set_Get_Controls."Set", "Action"=Motion_Translation_Module_Control."Velocity/Accel", "Error In"=w377, "Axis"=w381, "Table Stages"=w375) -> ("Error Out"=w380:errorcluster)  [unwired: 5 in, 1 out]
              }
              frame "Z Axis" {
              }
              frame "Y Axis" {
                n124 = Bundle By Name(cluster=w385, "Y Stage.Velocity"=w391) -> (w384:T11)
                n125 = call "XYZ Table Stage Module.vi"("Set/Get"=Set_Get_Controls."Set", "Action"=Motion_Translation_Module_Control."Velocity/Accel", "Error In"=w386, "Axis"=w390, "Table Stages"=w384) -> ("Error Out"=w389:errorcluster)  [unwired: 5 in, 1 out]
              }
            }
            n126 = call "Inline Wait.vi"("Error In"=w364, "milliseconds to wait"=u32 1000) -> ("Error Out"=w363:errorcluster)  [unwired: 9 in]
            n127 = case shown="Error" w363 {
              tunnel: [TRUE TRUE] -> w371
              frame No Error {
              }
              frame Error {
              }
            }
          }
        }
        n128 = case shown="Error" w16 {
          selector: w16 -> [w23 w24]
          tunnel: [w23 w24] -> w15
          tunnel: w14 -> [w22 w27]
          tunnel: [w21 w25] -> w13
          frame No Error {
            n129 = Delete From Array(array=w22, index=0) -> (array with subset deleted=w21:string[])  [unwired: 1 in, 1 out]
          }
          frame Error {
            n130 = Build Array (concatenate)("Error", w27) -> (w25:string[])
          }
        }
      }
    }
    frame Error {
    }
  }
  "error out" <- w1
